vi "HumanGetDeviceReference.vi"() -> (0 "ButtonBoard":T1, 1 "Aux Joy":T1, 3 "Driver Joy":T1)   [LabVIEW 2020]
uses:
  <vilib>/Rock Robotics/WPI/Joystick/WPI_JoystickDevRef.ctl
  <vilib>/Rock Robotics/WPI/Joystick/WPI_JoystickDeviceEnum.ctl
  <vilib>/Rock Robotics/WPI/Utilities/WPI_GetSetVariantRefNum.vi
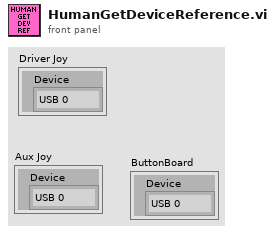
[diagram p1: front panel]
types:
  T1 = typedef "WPI_JoystickDevRef.ctl" = cluster{"Device":T2}
  T2 = typedef "WPI_JoystickDeviceEnum.ctl" = enum16{"USB 0", "USB 1", "USB 2", "USB 3", "USB 4", "USB 5"}
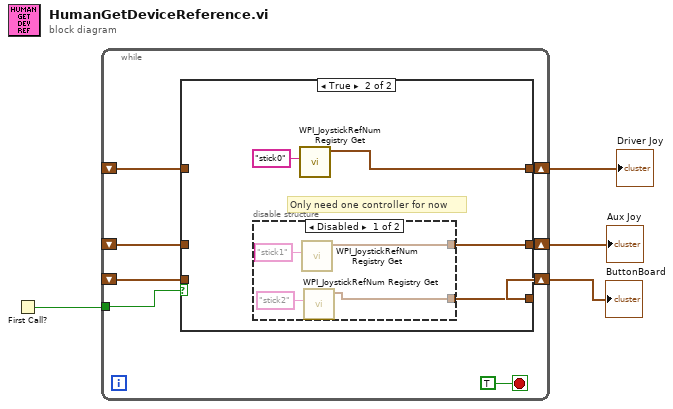
[diagram p0: block diagram]
diagram:
  n1 = First Call?() -> (First Call?: T/F=w2:bool)
  n2 = while {
    shift-right: [w10] -> w4
    shift-left: _ -> [w8]
    shift-right: [w9] -> w3
    shift-left: _ -> [w7]
    tunnel: w2 -> [w11]
    shift-right: [w6] -> w1
    shift-left: _ -> [w5]
    stop <- TRUE stop-if-true
    n3 = case shown="True" w11 {
      tunnel: [w15 w18] -> w10
      tunnel: [w14 w17] -> w9
      tunnel: w8 -> [w15 _]
      tunnel: w7 -> [w14 _]
      tunnel: [w13 w16] -> w6
      tunnel: w5 -> [w13 _]
      frame False {
      }
      frame True {
        # "Only need one controller for now"
        n4 = disable-structure shown="Disabled" {
          disable-tunnel: [w22 _] -> w17
          disable-tunnel: [w20 _] -> w16
          frame Disabled {
            n5 = call <vilib>:"WPI_JoystickRefNum Registry Get.vi"("refnum name"="stick1") -> ("JoystickDevRef"=w22:T1)  [unwired: 9 in, 1 out]
            n6 = call <vilib>:"WPI_JoystickRefNum Registry Get.vi"("refnum name"="stick2") -> ("JoystickDevRef"=w20:T1)  [unwired: 9 in, 1 out]
          }
          frame Enabled {
          }
        }
        n7 = call <vilib>:"WPI_JoystickRefNum Registry Get.vi"("refnum name"="stick0") -> ("JoystickDevRef"=w18:T1)  [unwired: 9 in, 1 out]
      }
    }
  }
  "Aux Joy" <- w3
  "Driver Joy" <- w4
  "ButtonBoard" <- w1
